vi "Periodic Tasks.vi"(8 "error in":errorcluster) -> ()   [LabVIEW 2016]
doc: "This VI runs in parallel to other tasks. It can contain as many user-defined periodic loops as you need. These can carry out PID or other sorts of timed response."
uses:
  Robot Global Data.vi
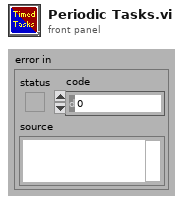
[diagram p1: front panel]
types:
  T1 = typedef "WPI_EncoderDevRef.ctl" = cluster{"DevStatus":errorcluster, "EncoderIndex":T2, "CounterIndex":T3, "DistancePerCount":dbl, "Decoding Type":T4}
  T2 = typedef "FPGA_EncoderIdx.ctl" = enum8{"Enc 0", "Enc 1", "Enc 2", "Enc 3", "Enc 4", "Enc 5", "Enc 6", "Enc 7", "Invalid"}
  T3 = typedef "FPGA_CounterCtrSystemIndex.ctl" = enum8{"Ctr 0", "Ctr 1", "Ctr 2", "Ctr 3", "Ctr 4", "Ctr 5", "Ctr 6", "Ctr 7", "Invalid"}
  T4 = typedef "WPI_EncoderType.ctl" = enum16{"1x", "2x", "4x"}
  T5 = typedef "WPI_MotorControlDeviceRef.ctl" = cluster{"DeviceStatus":errorcluster, "Type":T6, "PWM":cluster{"PWM Channel":T7, "DeadBand":T8}, "CAN":cluster{"Device Number":u8, "SetOutput VI Ref":variant, "GetOutput VI Ref":variant, "Enable VI Ref":variant, "Disable VI Ref":variant, "Data":variant}, "Invert":bool}
  T6 = typedef "WPI_MotorControlType.ctl" = enum16{"PWM", "CAN"}
  T7 = typedef "FPGA_DIOPWMChannel.ctl" = enum8{"PWM 0", "PWM 1", "PWM 2", "PWM 3", "PWM 4", "PWM 5", "PWM 6", "PWM 7", "PWM 8", "PWM 9", "PWM MXP 0", "PWM MXP 1", "PWM MXP 2", "PWM MXP 3", "PWM MXP 4", "PWM MXP 5", "PWM MXP 6", "PWM MXP 7", "PWM MXP 8", "PWM MXP 9", "Invalid"}
  T8 = typedef "WPI_PWMDeadband.ctl" = cluster{"Name":string, "maxPositivePwm":i32, "minPositivePwm":i32, "centerPwm":i32, "maxNegativePwm":i32, "minNegativePwm":i32, "angularRange":u16}
  T9 = cluster{"Distance (ft)":dbl, "Score":dbl, "Normalized":cluster{"Center":cluster{dbl, dbl}, "Rectangle":cluster{"Numeric":dbl, "Numeric 2":dbl, "Numeric 3":dbl, "Numeric 5":dbl}}, "Pixels":cluster{"Center":cluster{dbl, dbl}, "Rectangle":cluster{"Numeric":dbl, "Numeric 2":dbl, "Numeric 3":dbl, "Numeric 5":dbl}}}
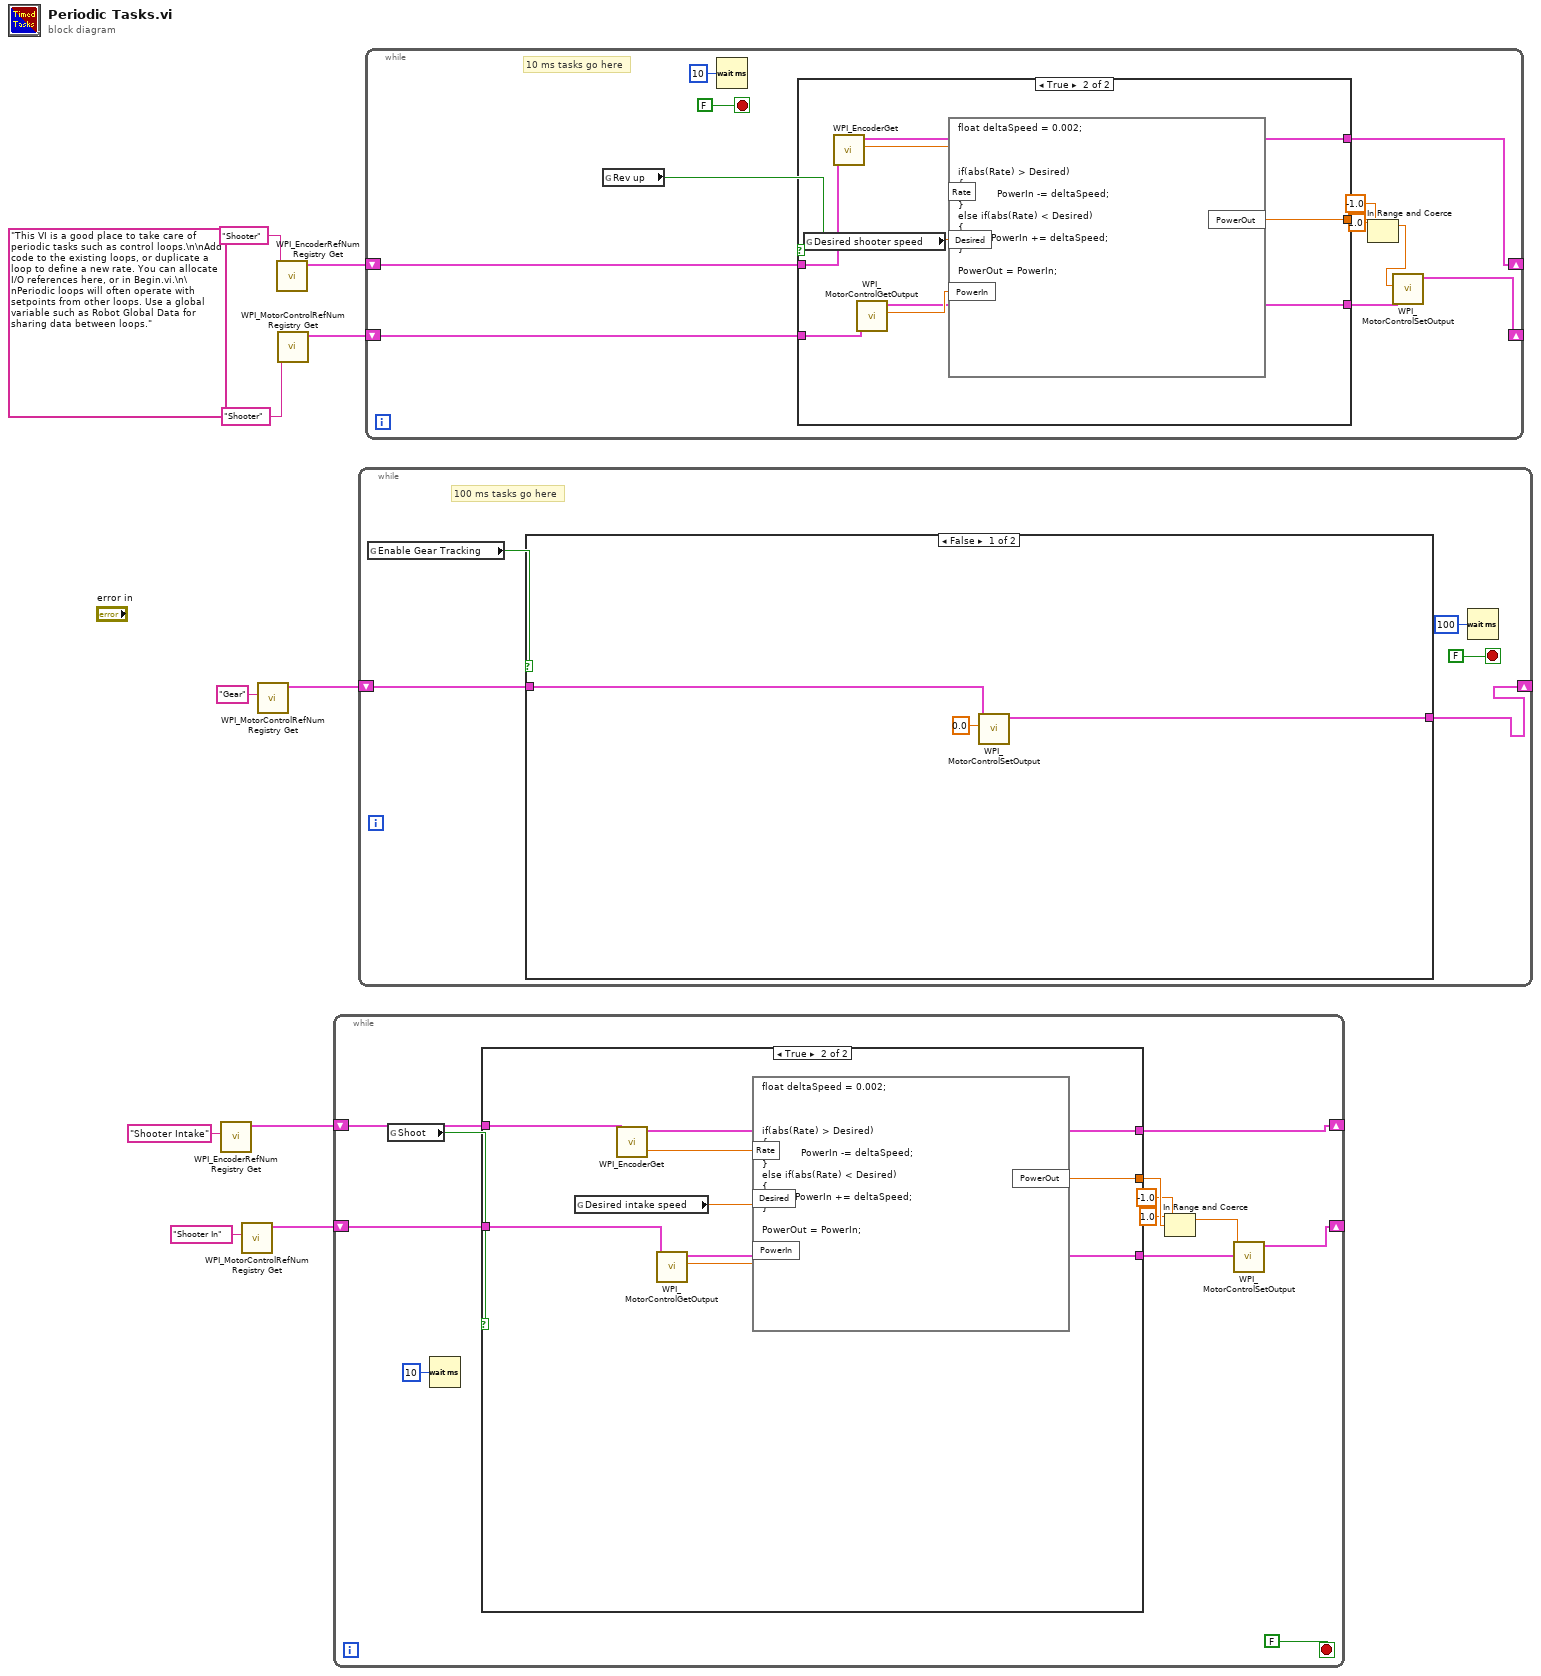
[diagram p0: block diagram]
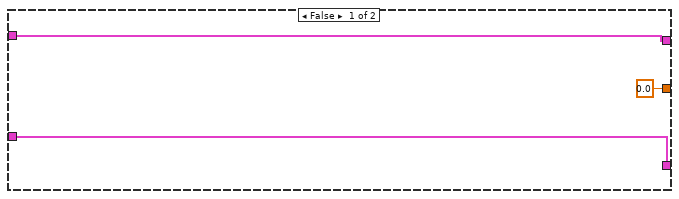
[diagram p2: hidden frame]
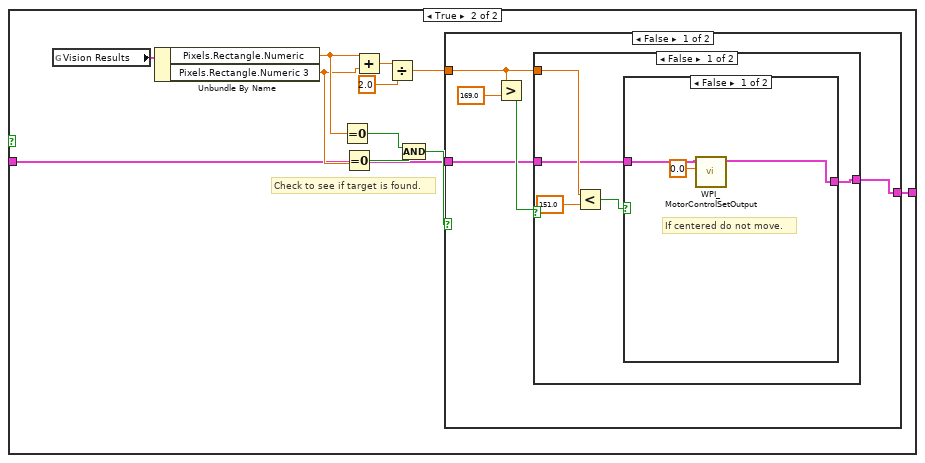
[diagram p3: hidden frame]
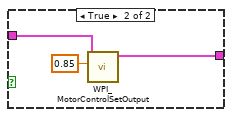
[diagram p4: hidden frame]
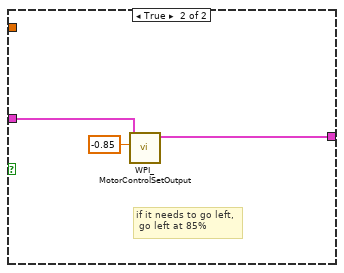
[diagram p5: hidden frame]
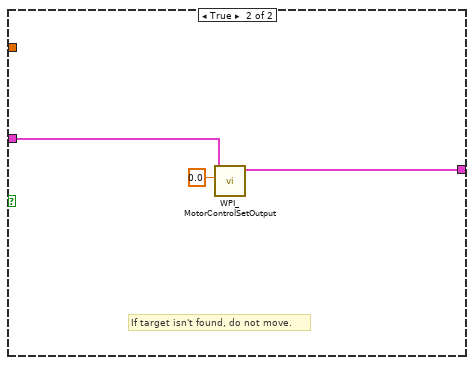
[diagram p6: hidden frame]
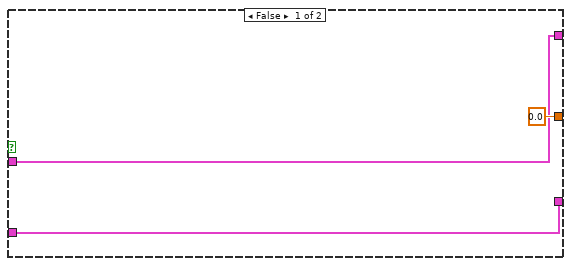
[diagram p7: hidden frame]
diagram:
  (unwired) "This VI is a good place to take care of periodic tasks such as control loops.\n\nAdd code to the existing loops, or duplicate a loop to define a new rate. You can allocate I/O references here, or in Begin.vi.\n\nPeriodic loops will often operate with setpoints from other loops. Use a global variable such as Robot Global Data for sharing data between loops."
  n1 = call <vilib>:"WPI_EncoderRefNum Registry Get.vi"("refnum name"="Shooter Intake") -> ("EncoderDevRef"=w5:T1)  [unwired: 9 in, 1 out]
  n2 = call <vilib>:"WPI_MotorControlRefNum Registry Get.vi"("refnum name"="Shooter In") -> ("MotorControlDevRef"=w7:T5)  [unwired: 9 in, 1 out]
  n3 = call <vilib>:"WPI_MotorControlRefNum Registry Get.vi"("refnum name"="Gear") -> ("MotorControlDevRef"=w9:T5)  [unwired: 9 in, 1 out]
  n4 = call <vilib>:"WPI_EncoderRefNum Registry Get.vi"("refnum name"="Shooter") -> ("EncoderDevRef"=w2:T1)  [unwired: 9 in, 1 out]
  n5 = call <vilib>:"WPI_MotorControlRefNum Registry Get.vi"("refnum name"="Shooter") -> ("MotorControlDevRef"=w1:T5)  [unwired: 9 in, 1 out]
  n6 = while {
    shift-right: [w14] -> _
    shift-left: w7 -> [w21]
    shift-right: [w12] -> _
    shift-left: w5 -> [w13]
    stop <- FALSE stop-if-true
    n7 = global read "Robot Global Data.vi" "Shoot"() -> (w22:bool)
    n8 = Wait (ms)(milliseconds to wait=u32 10) -> ()  [unwired: 1 out]
    n9 = case shown="True" w22 {
      tunnel: w21 -> [w24 w32]
      tunnel: [0.0 ("PowerOut") w30] -> w19
      tunnel: [w24 w29] -> w15
      tunnel: w13 -> [w23 w27]
      tunnel: [w23 w26] -> w12
      frame False {
      }
      frame True {
        n10 = global read "Robot Global Data.vi" "Desired intake speed"() -> (w31:dbl)
        n11 = call <vilib>:"WPI_EncoderGet.vi"("EncoderDevRef"=w27) -> ("EncoderDevRef"=w26:T1, "Rate"=w28:dbl)  [unwired: 5 in, 4 out]
        n12 = call <vilib>:"WPI_MotorControlGetOutput.vi"("MotorControlDevRef"=w32) -> ("Output"=w33:dbl, "MotorControlDevRef"=w29:T5)  [unwired: 8 in, 1 out]
        n13 = formula code="float deltaSpeed = 0.002;\n\n\n\nif(abs(Rate) > Desired)\n{\n             PowerIn -= deltaSpeed;\n}\nelse if(abs(Rate) < Desired)\n{\n           PowerIn += deltaSpeed;\n}\n\nPowerOut = PowerIn;"("Rate"=w28, "Desired"=w31, "PowerIn"=w33) -> ("PowerOut"=w30:dbl)
      }
    }
    n14 = In Range and Coerce(upper limit=1.0, x=w19, lower limit=-1.0) -> (coerced(x)=w16:dbl)  [unwired: 1 out]
    n15 = call <vilib>:"WPI_MotorControlSetOutput.vi"("Output"=w16, "MotorControlDevRef"=w15) -> ("MotorControlDevRef"=w14:T5)  [unwired: 7 in, 2 out]
  }
  n16 = while {
    shift-right: [w34] -> _
    shift-left: w9 -> [w35]
    stop <- FALSE stop-if-true
    # "100 ms tasks go here"
    n17 = global read "Robot Global Data.vi" "Enable Gear Tracking"() -> (w36:bool)
    n18 = case shown="False" w36 {
      tunnel: w35 -> [w41 w44]
      tunnel: [w40 w43] -> w34
      frame False {
        n19 = call <vilib>:"WPI_MotorControlSetOutput.vi"("Output"=0.0, "MotorControlDevRef"=w41) -> ("MotorControlDevRef"=w40:T5)  [unwired: 7 in, 2 out]
      }
      frame True {
        # "Check to see if target is found."
        n20 = global read "Robot Global Data.vi" "Vision Results"() -> (w52:T9)
        n21 = Unbundle By Name(w52) -> ("Pixels.Rectangle.Numeric"=w51:dbl, "Pixels.Rectangle.Numeric 3"=w50:dbl)
        n22 = Equal To 0?(x=w51) -> (x = 0?=w49:bool)
        n23 = Equal To 0?(x=w50) -> (x = 0?=w48:bool)
        n24 = Add(x=w51, y=w50) -> (x+y=w47:dbl)
        n25 = Divide(x=w47, y=2.0) -> (x/y=w42:dbl)
        n26 = Compound Arithmetic op=AND(w49, w48) -> (w45:bool)
        n27 = case shown="False" w45 {
          tunnel: w44 -> [w55 w73]
          tunnel: [w54 w72] -> w43
          tunnel: w42 -> [w53 _]
          frame False {
            n28 = Greater?(x=w53, y=169.0) -> (0:w56:bool)
            n29 = case shown="False" w56 {
              tunnel: w55 -> [w59 w70]
              tunnel: [w58 w69] -> w54
              tunnel: w53 -> [w61 _]
              frame False {
                n30 = Less?(x=w61, y=151.0) -> (x < y?=w60:bool)
                n31 = case shown="False" w60 {
                  tunnel: w59 -> [w64 w67]
                  tunnel: [w63 w66] -> w58
                  frame False {
                    # "If centered do not move."
                    n32 = call <vilib>:"WPI_MotorControlSetOutput.vi"("Output"=0.0, "MotorControlDevRef"=w64) -> ("MotorControlDevRef"=w63:T5)  [unwired: 7 in, 2 out]
                  }
                  frame True {
                    n33 = call <vilib>:"WPI_MotorControlSetOutput.vi"("Output"=0.85, "MotorControlDevRef"=w67) -> ("MotorControlDevRef"=w66:T5)  [unwired: 7 in, 2 out]
                  }
                }
              }
              frame True {
                # "if it needs to go left,\n go left at 85%"
                n34 = call <vilib>:"WPI_MotorControlSetOutput.vi"("Output"=-0.85, "MotorControlDevRef"=w70) -> ("MotorControlDevRef"=w69:T5)  [unwired: 7 in, 2 out]
              }
            }
          }
          frame True {
            # "If target isn't found, do not move."
            n35 = call <vilib>:"WPI_MotorControlSetOutput.vi"("Output"=0.0, "MotorControlDevRef"=w73) -> ("MotorControlDevRef"=w72:T5)  [unwired: 7 in, 2 out]
          }
        }
      }
    }
    n36 = Wait (ms)(milliseconds to wait=u32 100) -> ()  [unwired: 1 out]
  }
  n37 = while {
    shift-right: [w75] -> _
    shift-left: w2 -> [w76]
    shift-right: [w77] -> _
    shift-left: w1 -> [w83]
    stop <- FALSE stop-if-true
    # "10 ms tasks go here"
    n38 = global read "Robot Global Data.vi" "Rev up"() -> (w84:bool)
    n39 = Wait (ms)(milliseconds to wait=u32 10) -> ()  [unwired: 1 out]
    n40 = case shown="True" w84 {
      tunnel: w83 -> [w89 w95]
      tunnel: [0.0 ("PowerOut") w94] -> w82
      tunnel: [w89 w93] -> w78
      tunnel: w76 -> [w87 w92]
      tunnel: [w87 w90] -> w75
      frame False {
      }
      frame True {
        n41 = global read "Robot Global Data.vi" "Desired shooter speed"() -> (w97:dbl)
        n42 = call <vilib>:"WPI_EncoderGet.vi"("EncoderDevRef"=w92) -> ("Distance"=w91:dbl, "EncoderDevRef"=w90:T1)  [unwired: 5 in, 4 out]
        n43 = call <vilib>:"WPI_MotorControlGetOutput.vi"("MotorControlDevRef"=w95) -> ("Output"=w96:dbl, "MotorControlDevRef"=w93:T5)  [unwired: 8 in, 1 out]
        n44 = formula code="float deltaSpeed = 0.002;\n\n\n\nif(abs(Rate) > Desired)\n{\n             PowerIn -= deltaSpeed;\n}\nelse if(abs(Rate) < Desired)\n{\n           PowerIn += deltaSpeed;\n}\n\nPowerOut = PowerIn;"("Rate"=w91, "Desired"=w97, "PowerIn"=w96) -> ("PowerOut"=w94:dbl)
      }
    }
    n45 = In Range and Coerce(upper limit=1.0, x=w82, lower limit=-1.0) -> (coerced(x)=w79:dbl)  [unwired: 1 out]
    n46 = call <vilib>:"WPI_MotorControlSetOutput.vi"("Output"=w79, "MotorControlDevRef"=w78) -> ("MotorControlDevRef"=w77:T5)  [unwired: 7 in, 2 out]
  }
